vi "On-Off Epoxy.vi"   [LabVIEW 2021]
uses:
  Classes/Controller/Controller.lvclass
  Classes/Controller/Dispenser/Dispenser.lvclass
  C:/Users/HEP/Documents/GitHub/UCSB-Gantry-HEP/Classes/Controller/Controller.lvclass
  C:/Users/HEP/Documents/GitHub/UCSB-Gantry-HEP/Classes/Controller/Dispenser/Dispenser.lvclass
types:
  T1 = typedef "Controller.lvclass/Controllers.ctl" = cluster{"I-O.lvclass":refnum<class "I-O.lvclass">, "Gantry":refnum<k24>, "Dispenser":refnum<visa-resource-name>}
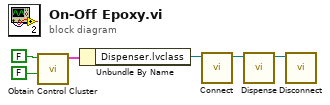
[diagram p0: block diagram]
diagram:
  n1 = call "Obtain Control Cluster.vi"("I/O"=FALSE, "Motion"=FALSE) -> ("Control Out"=w4:T1)  [unwired: 9 in]
  n2 = Unbundle By Name(w4) -> ("Dispenser.lvclass"=w3:refnum<class "Dispenser.lvclass">)
  n3 = call-dynamic "Connect.vi"("Controller in"=w3) -> ("Controller out"=w6:refnum<class "Dispenser.lvclass">)  [unwired: 9 in, 1 out]
  n4 = call "Dispense.vi"("Dispenser In"=w6) -> ("Dispenser Out"=w5:refnum<visa-resource-name>)  [unwired: 9 in, 1 out]
  n5 = call-dynamic "Disconnect.vi"("Controller in"=w5) -> ()  [unwired: 9 in, 1 out]
